vi "DownloadPackageFromNevstopFTP.vi"(7 "ftp":T1={"address"="vipm.nevstop.top", "remote port (21)"=1986, "userName"="anonymous", "passWord"="anonymous"}, 8 "error in (no error)":errorcluster, 11 "CommandLine":string="Communicable-State-Machine") -> (0 "error out":errorcluster, 2 "test details":string="FTP package Candidates:", 3 "localdir":path)   [LabVIEW 2017, in "_Try Beta Version of CSMF.lvlib"]
uses:
  _Try Beta Version of CSMF.lvlib
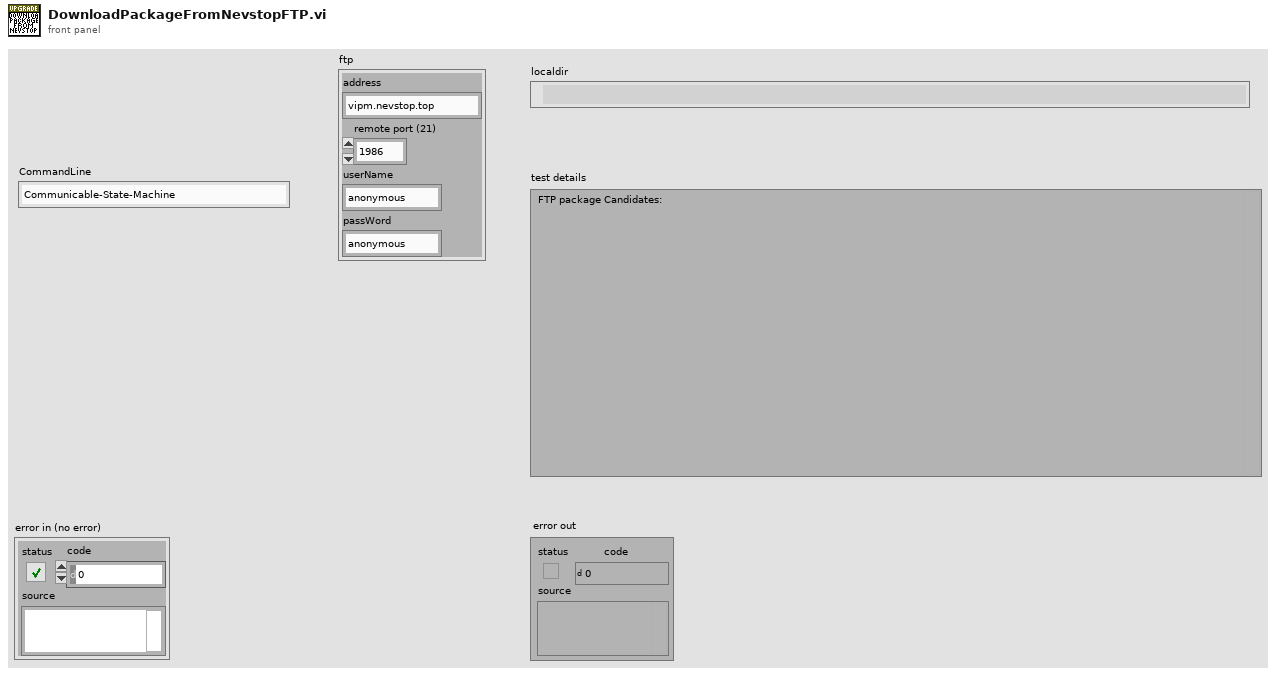
[diagram p1: front panel]
types:
  T1 = cluster{"address":string, "remote port (21)":u16, "userName":string, "passWord":string}
  T2 = typedef "FTP_UpgradeCSMF.lvlib/FTP.lvclass/Dir-File Info.ctl" = cluster{"Name":string, "Modify Timestamp":timestamp, "Dir-File Type":T3, "Unique Id":string, "Permissions":string, "Unix Mode":u16, "Owner":string, "Group":string, "FileSize":i64}
  T3 = typedef "FTP_UpgradeCSMF.lvlib/FTP.lvclass/Dir-File Type.ctl" = enum16{"File", "Listed Directory", "Parent Directory", "Directory", "Unknown"}
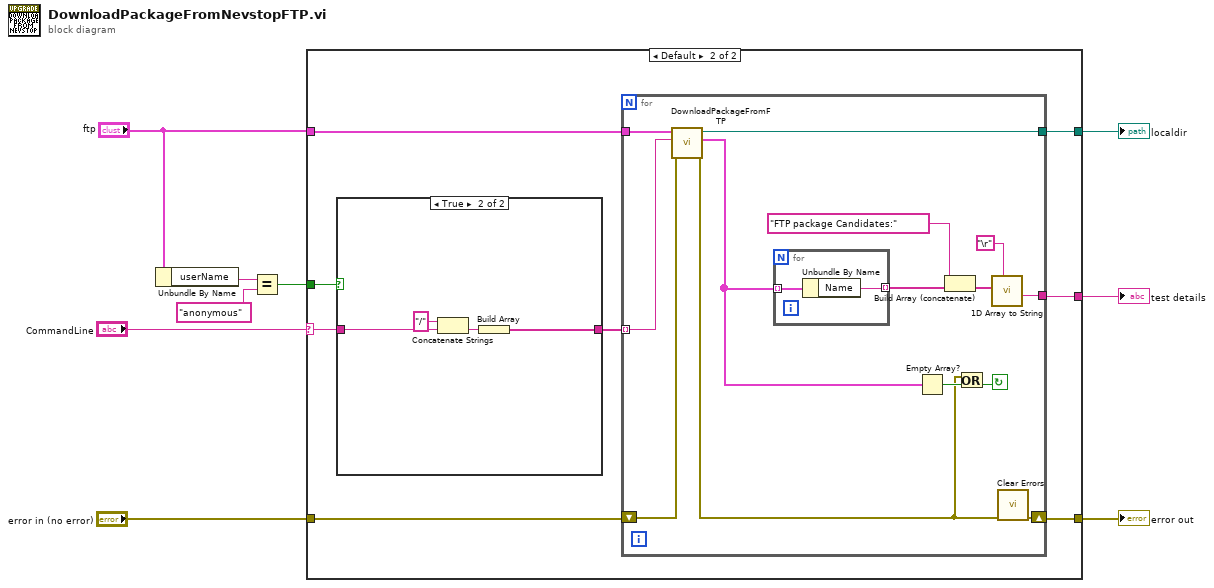
[diagram p0: block diagram]
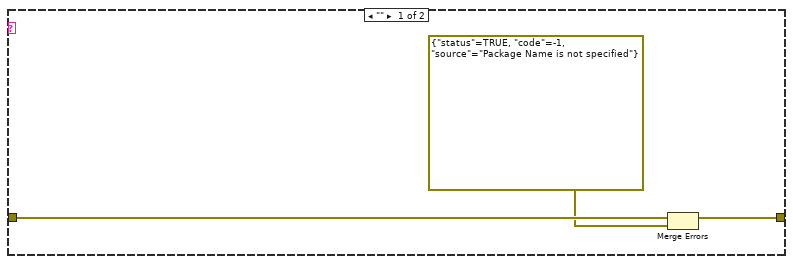
[diagram p2: hidden frame]
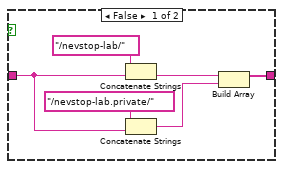
[diagram p3: hidden frame]
diagram:
  n1 = Unbundle By Name("ftp") -> ("userName"=w3:string)
  n2 = Equal?(x=w3, y="anonymous") -> (x = y?=w5:bool)
  n3 = case shown="Default" "CommandLine" {
    selector: "CommandLine" -> [_ w14]
    tunnel: [_ w20] -> w9
    tunnel: "ftp" -> [_ w19]
    tunnel: "error in (no error)" -> [w12 w18]
    tunnel: [_ w17] -> w1
    tunnel: [w11 w16] -> w7
    tunnel: w5 -> [_ w15]
    frame "" {
      n4 = Merge Errors(w12, errorcluster {"status"=TRUE, "code"=-1, "source"="Package Name is not specified"} ("error in")) -> (w11:errorcluster)
    }
    frame Default {
      n5 = case shown="True" w15 {
        tunnel: w14 -> [w37 w46]
        tunnel: [w40 w43] -> w13
        frame False {
          n6 = Concatenate Strings("/nevstop-lab/" ("RemoteDirectory"), w37) -> (w41:string)
          n7 = Concatenate Strings("/nevstop-lab.private/" ("RemoteDirectory"), w37) -> (w38:string)
          n8 = Build Array(w41, w38) -> (w40:string[])
        }
        frame True {
          n9 = Concatenate Strings("/" ("string"), w46) -> (w45:string)
          n10 = Build Array(w45) -> (w43:string[])
        }
      }
      n11 = for {
        tunnel: [w32] -> w20
        tunnel: w19 -> [w31]
        tunnel: [w29] -> w17
        tunnel: w13 -> [w26] mode=indexing
        shift-right: [w24] -> w16
        shift-left: w18 -> [w30]
        stop <- w22 continue-if-true
        n12 = call "DownloadPackageFromFTP.vi"("error in (no error)"=w30, "RemoteDirectory"=w26, "ftp"=w31) -> ("error out"=w21:errorcluster, "candidates"=w25:T2[], "localdir"=w29:path)  [unwired: 5 in, 1 out]
        n13 = for {
          tunnel: [w35] -> w34 mode=indexing
          tunnel: w25 -> [w36] mode=indexing
          n14 = Unbundle By Name(w36) -> ("Name"=w35:string)
        }
        n15 = Empty Array?(array=w25) -> (empty?=w23:bool)
        n16 = Build Array (concatenate)("FTP package Candidates:" ("Name"), w34) -> (w28:string[])
        n17 = Or(x=w21, y=w23) -> (x .or. y?=w22:bool)
        n18 = call "1D Array to String.vi"("delimiter (Tab)"="\r", "Array of Strings"=w28) -> ("delimited string"=w32:string)  [unwired: 9 in]
        n19 = call <vilib>:"Clear Errors.vi"("error in (no error)"=w21) -> ("error out"=w24:errorcluster)  [unwired: 5 in, 1 out]
      }
    }
  }
  "test details" <- w9
  "error out" <- w7
  "localdir" <- w1
